vi "CheckCorrectInputs.vi"(9 "Step":dbl caption="Krok", 10 "Max":dbl caption="Koneèná hodnota", 11 "Min":dbl caption="Poèáteèní hodnota") -> (3 "x .or. y?":bool)   [LabVIEW 2021]
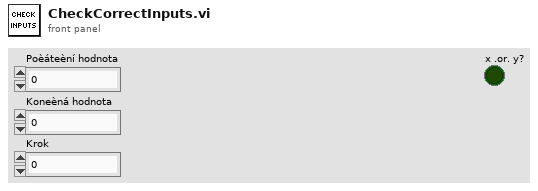
[diagram p1: front panel]
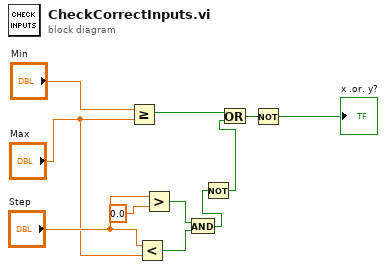
[diagram p0: block diagram]
diagram:
  n1 = Greater Or Equal?(x="Min", y="Max") -> (x >= y?=w8:bool)
  n2 = Less?(x="Step", y="Max") -> (x < y?=w6:bool)
  n3 = Greater?(x="Step", y=0.0) -> (0:w7:bool)
  n4 = And(x=w7, y=w6) -> (x .and. y?=w5:bool)
  n5 = Not(x=w5) -> (.not. x?=w4:bool)
  n6 = Or(x=w8, y=w4) -> (x .or. y?=w2:bool)
  n7 = Not(x=w2) -> (.not. x?=→"x .or. y?":bool)
